vi "Database-GetPrevStatus.vi"(8 "error in":errorcluster, 9 "Serial":string[](array[string]), 10 "Refs":string[](array[string]), 11 "Idx":i32) -> (0 "error out":errorcluster, 2 "Status":i8)   [LabVIEW 2016]
doc: "Go to DB->WriteStationValues action\nReturn boolean flag to show if data was saved to DB successfully\n\nWabco 2017 All right reserved\nAuthor: maciej.szupienko@wabco-auto.com"
uses:
  Database.Action.ctl
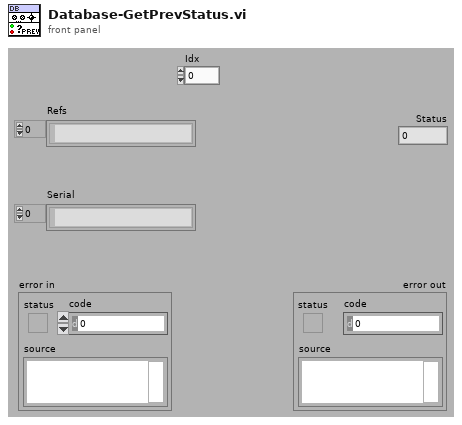
[diagram p1: front panel]
types:
  T1 = typedef "Database.Action.ctl" = enum32{"idle", "constructor", "destructor", "--- DB ---", "Setup", "Disconnect", "Connect", "GetAllStatuses"}
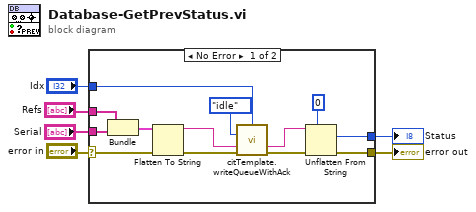
[diagram p0: block diagram]
diagram:
  n1 = case shown="No Error" "error in" {
    selector: "error in" -> [w17 w20]
    tunnel: [w15 w20] -> w5
    tunnel: "Idx" -> [w19 _]
    tunnel: "Serial" -> [w12 _]
    tunnel: "Refs" -> [w11 _]
    tunnel: [w7 _] -> w3
    frame No Error {
      n2 = Bundle("Refs"=w11, "Serial"=w12) -> (w13:cluster{"Refs":string[], "Serial":string[]})  [unwired: 1 in]
      n3 = Flatten To String(anything=w13, error in (no error)=w17) -> (data string=w9:string, error out=w16:errorcluster)  [unwired: 2 in, 1 out]
      n4 = call "citTemplate.writeQueueWithAck.vi"("instance (0)"=w19, "event in"=Database.Action."idle" ("Action"), "(flatten) data in"=w9, "error in (no error)"=w16) -> ("notification data"=w14:string, "error out"=w18:errorcluster)  [unwired: 9 in, 1 out]
      n5 = Unflatten From String(type=i8 0, binary string=w14, error in (no error)=w18) -> (value=w7:i8, error out=w15:errorcluster)  [unwired: 2 in, 1 out]
    }
    frame Error {
    }
  }
  "error out" <- w5
  "Status" <- w3
